vi "Consume Packet Token.vi"(11 "Packet Parser In":T2) -> (0 "End?":bool, 1 "Value":i32, 2 "Type":T1, 3 "Packet Parser":T2)   [LabVIEW 2022 SP3, in "AoC22.lvlib"]
uses:
  AoC22.lvlib
  Packet Parser.ctl
  Packet Token.ctl
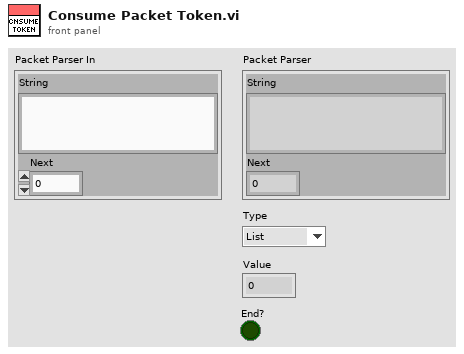
[diagram p1: front panel]
types:
  T1 = typedef "AoC22.lvlib/Packet Token.ctl" = enum16{"List", "End List", "Value", "Comma"}
  T2 = typedef "AoC22.lvlib/Packet Parser.ctl" = cluster{"String":string, "Next":i32}
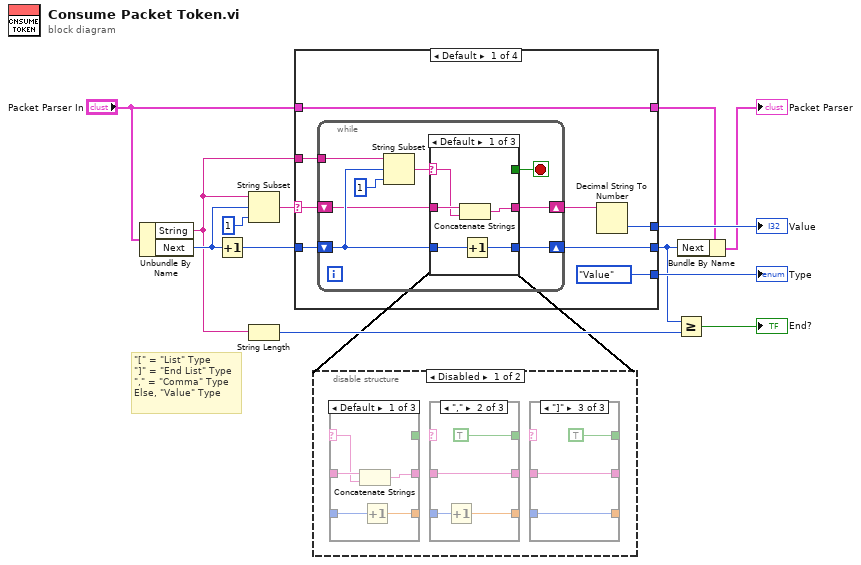
[diagram p0: block diagram]
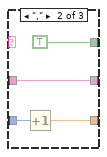
[diagram p2: hidden frame]
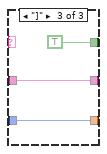
[diagram p3: hidden frame]
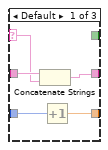
[diagram p4: hidden frame]
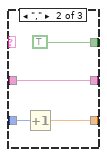
[diagram p5: hidden frame]
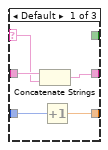
[diagram p6: hidden frame]
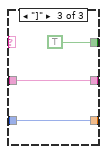
[diagram p7: hidden frame]
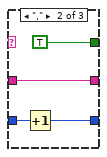
[diagram p9: hidden frame]
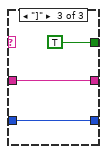
[diagram p10: hidden frame]
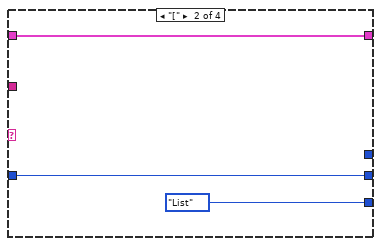
[diagram p11: hidden frame]
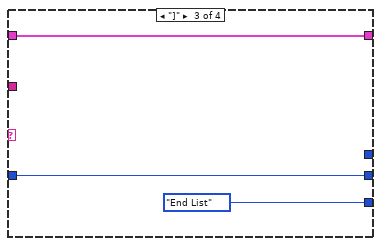
[diagram p12: hidden frame]
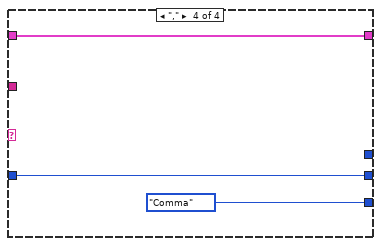
[diagram p13: hidden frame]
diagram:
  # "\"[\" = \"List\" Type\n\"]\" = \"End List\" Type\n\",\" = \"Comma\" Type\nElse, \"Value\" Type"
  n1 = Unbundle By Name("Packet Parser In") -> ("String"=w4:string, "Next"=w9:i32)
  n2 = Increment(x=w9) -> (x+1=w8:i32)
  n3 = String Subset(string=w4, offset (0)=w9, length (rest)=1 ("length (rest)")) -> (substring=w11:string)
  n4 = String Length(string=w4) -> (length=w3:i32)
  n5 = case shown="Default" w11 {
    selector: w11 -> [w21 _ _ _]
    tunnel: "Packet Parser In" -> [w15 w42 w45 w50]
    tunnel: w8 -> [w20 w44 w47 w49]
    tunnel: [w15 w42 w45 w50] -> w6
    tunnel: [Packet_Token."Value" ("Packet Token") Packet_Token."List" ("Packet Token") Packet_Token."End List" ("Packet Token") Packet_Token."Comma" ("Packet Token")] -> w7
    tunnel: [w18 _ _ _] -> w13
    tunnel: w4 -> [w16 _ _ _]
    tunnel: [w14 w44 w47 w49] -> w1
    frame Default {
      n6 = while {
        shift-right: [w23] -> w19
        shift-left: w21 -> [w24]
        shift-right: [w25] -> w14
        shift-left: w20 -> [w26]
        tunnel: w16 -> [w29]
        stop <- w22 stop-if-true
        n7 = String Subset(string=w29, offset (0)=w26, length (rest)=1 ("length (rest)")) -> (substring=w27:string)
        n8 = case shown="Default" w27 {
          selector: w27 -> [w33 _ _]
          tunnel: w26 -> [w31 w38 w40]
          tunnel: [w30 w37 w40] -> w25
          tunnel: w24 -> [w34 w36 w41]
          tunnel: [w32 w36 w41] -> w23
          tunnel: [_ TRUE TRUE] -> w22
          frame Default {
            n9 = Concatenate Strings(w34, w33) -> (w32:string)
            n10 = Increment(x=w31) -> (x+1=w30:i32)
          }
          frame "," {
            n11 = Increment(x=w38) -> (x+1=w37:i32)
          }
          frame "]" {
          }
        }
      }
      n12 = Decimal String To Number(string=w19) -> (number=w18:i32)  [unwired: 2 in, 1 out]
    }
    frame "[" {
    }
    frame "]" {
    }
    frame "," {
    }
  }
  "Value" <- w13
  "Type" <- w7
  n13 = disable-structure shown="Disabled" {
    frame Disabled {
      n14 = case shown="Default" {
        selector: _ -> [w54 _ _]
        tunnel: _ -> [w52 w59 w61]
        tunnel: [w51 w58 w61] -> _
        tunnel: _ -> [w55 w57 w62]
        tunnel: [w53 w57 w62] -> _
        tunnel: [_ TRUE TRUE] -> _
        frame Default {
          n15 = Concatenate Strings(w55, w54) -> (w53:string)
          n16 = Increment(x=w52) -> (x+1=w51:dbl)
        }
        frame "," {
          n17 = Increment(x=w59) -> (x+1=w58:dbl)
        }
        frame "]" {
        }
      }
      n18 = case shown="\",\"" {
        selector: _ -> [w78 _ _]
        tunnel: _ -> [w76 w83 w85]
        tunnel: [w75 w82 w85] -> _
        tunnel: _ -> [w79 w81 w86]
        tunnel: [w77 w81 w86] -> _
        tunnel: [_ TRUE TRUE] -> _
        frame Default {
          n19 = Concatenate Strings(w79, w78) -> (w77:string)
          n20 = Increment(x=w76) -> (x+1=w75:dbl)
        }
        frame "," {
          n21 = Increment(x=w83) -> (x+1=w82:dbl)
        }
        frame "]" {
        }
      }
      n22 = case shown="\"]\"" {
        selector: _ -> [w66 _ _]
        tunnel: _ -> [w64 w71 w73]
        tunnel: [w63 w70 w73] -> _
        tunnel: _ -> [w67 w69 w74]
        tunnel: [w65 w69 w74] -> _
        tunnel: [_ TRUE TRUE] -> _
        frame Default {
          n23 = Concatenate Strings(w67, w66) -> (w65:string)
          n24 = Increment(x=w64) -> (x+1=w63:dbl)
        }
        frame "," {
          n25 = Increment(x=w71) -> (x+1=w70:dbl)
        }
        frame "]" {
        }
      }
    }
    frame Enabled {
    }
  }
  n26 = Greater Or Equal?(x=w1, y=w3) -> (x >= y?=→"End?":bool)
  n27 = Bundle By Name(cluster=w6, "Next"=w1) -> (→"Packet Parser":T2)
